vi "cal_joints padrao.vi"(11 "Joints":dbl[][](array[numeric])) -> ()   [LabVIEW 2016]
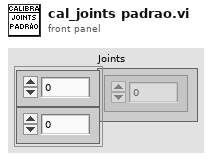
[diagram p1: front panel]
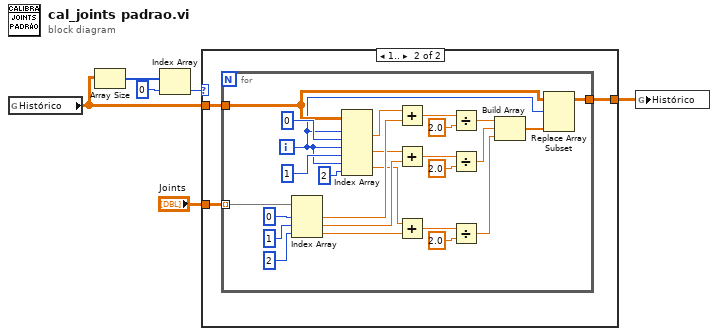
[diagram p0: block diagram]
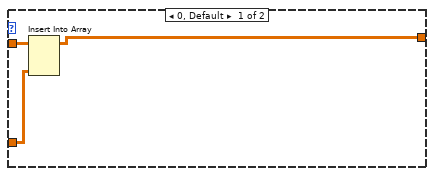
[diagram p2: hidden frame]
diagram:
  n1 = global read "historico_calibraçcao.vi" "Histórico"() -> (w3:dbl[][])
  n2 = Array Size(array=w3) -> (size(s)=w6:i32[])
  n3 = Index Array(array=w6, index=0) -> (element=w5:i32)
  n4 = case shown="1.." w5 {
    tunnel: w3 -> [w9 w11]
    tunnel: "Joints" -> [w8 w12]
    tunnel: [w7 w10] -> w1
    frame 0, Default {
      n5 = Insert Into Array(array=w9, new element=w8) -> (w7:dbl[][])  [unwired: 2 in]
    }
    frame 1.. {
      n6 = for {
        tunnel: w12 -> [w35] mode=indexing
        tunnel: w11 -> [w16]
        tunnel: [w13] -> w10
        i -> [w14]
        n7 = Index Array(array=w35, index #1=0 ("index"), index #2=1 ("index"), index #3=2 ("index")) -> (element #1=w30:dbl, element #2=w26:dbl, element #3=w24:dbl)
        n8 = Index Array(array=w16, index (row) #1=w14, index (col) #1=0 ("disabled index (col)"), index (row) #2=w14, index (col) #2=1 ("disabled index (col)"), index (row) #3=w14, index (col) #3=2 ("disabled index (col)")) -> (element #1=w31:dbl, element #2=w27:dbl, element #3=w25:dbl)
        n9 = Add(x=w31, y=w30) -> (x+y=w29:dbl)
        n10 = Add(x=w27, y=w26) -> (x+y=w23:dbl)
        n11 = Add(x=w25, y=w24) -> (x+y=w21:dbl)
        n12 = Divide(x=w29, y=2.0) -> (x/y=w19:dbl)
        n13 = Divide(x=w23, y=2.0) -> (x/y=w18:dbl)
        n14 = Divide(x=w21, y=2.0) -> (x/y=w17:dbl)
        n15 = Build Array(w19, w18, w17) -> (w15:dbl[])
        n16 = Replace Array Subset(array=w16, new element=w15, index (row)=w14) -> (w13:dbl[][])  [unwired: 1 in]
      }
    }
  }
  n17 = global write "historico_calibraçcao.vi" "Histórico"(w1) -> ()
